vi "Import Routing and Faulting Custom Device.vi"(8 "error in (no error)":errorcluster, 10 "Path":path, 11 "Routing and Faulting Custom Device Ref in":T1 format="%.0x") -> (0 "error out":errorcluster, 3 "Routing and Faulting Custom Device Ref out":T1 format="%.0x")   [LabVIEW 2017, in "Routing and Faulting Scripting.lvlib"]
uses:
  Routing and Faulting Scripting.lvlib
  <vilib>/NI Veristand/Custom Device API/Custom Device Item Ref.ctl
  Utility/RaF Pre-Import Action.vi
  <vilib>/NI/NI VeriStand Custom Device Import and Export Tool/ImportExport.lvlib
  <vilib>/NI VeriStand/Custom Device API/Custom Device API.lvlib
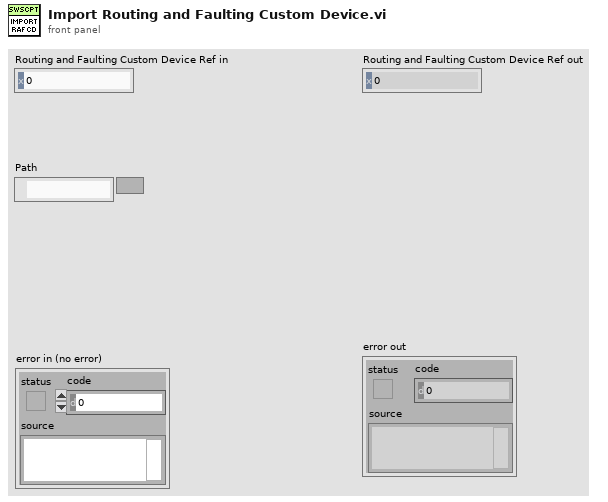
[diagram p1: front panel]
types:
  T1 = typedef "Custom Device API.lvlib/Custom Device Item Ref.ctl" = u64
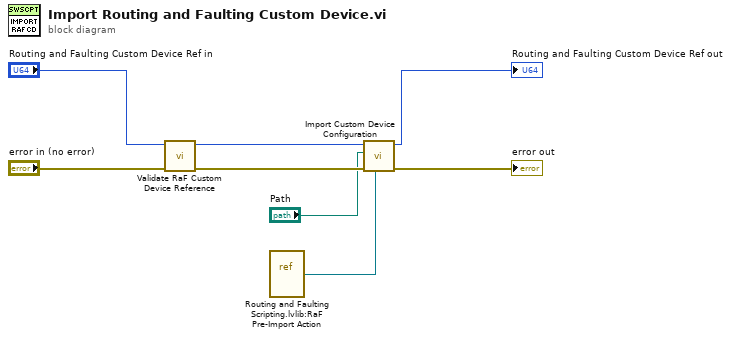
[diagram p0: block diagram]
diagram:
  n1 = call "Validate RaF Custom Device Reference.vi"("error in (no error)"="error in (no error)", "Routing and Faulting Custom Device Ref in"="Routing and Faulting Custom Device Ref in") -> ("error out"=w4:errorcluster, "Routing and Faulting Custom Device Ref out"=w5:T1)  [unwired: 8 in]
  n2 = vi-ref "Routing and Faulting Scripting.lvlib:RaF Pre-Import Action.vi"() -> (w6:refnum<vi>)
  n3 = call <vilib>:"Import Custom Device Configuration.vi"("Pre-Import Action"=w6, "error in (no error)"=w4, "Path"="Path", "NodeID"=w5) -> ("error out"=→"error out":errorcluster, "NodeID out"=→"Routing and Faulting Custom Device Ref out":u64)  [unwired: 5 in, 1 out]
